vi "Encode String.vi"(10 "String":string, 11 "URI-Component.Path":refnum<class "URI-Component.Path.lvclass">) -> (2 "Encoded String":string)   [LabVIEW 2013, in "openURI.lvlib" / "URI-Component.Path.lvclass"]
uses:
  URI-Component.Path.lvclass
  utilities/isHEXDigit.vi
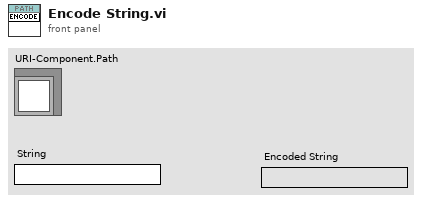
[diagram p1: front panel]
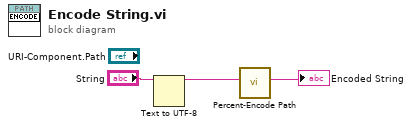
[diagram p0: block diagram]
diagram:
  n1 = Text to UTF-8(11:"String") -> (3:w1:string)  [unwired: 1 in, 1 out]
  n2 = call "Percent-Encode Path.vi"("Path"=w1) -> ("Pct-Encoded Path"=→"Encoded String":string)  [unwired: 10 in]
